vi "WriteScope.vi"(3 "error in (no error)":errorcluster caption="错误输入（无错误）", 4 "本次文件名":string, 5 "report in":refnum<class "NI_report.lvclass"> caption="报表输入") -> (0 "error out":errorcluster caption="错误输出", 2 "report out":refnum<class "NI_report.lvclass"> caption="报表输出")   [LabVIEW 2018]
uses:
  <vilib>/Utility/NIReport.llb/NI_report.lvclass
  ReportItem.ctl
  Init/AllPath.vi
  Reslut.vi
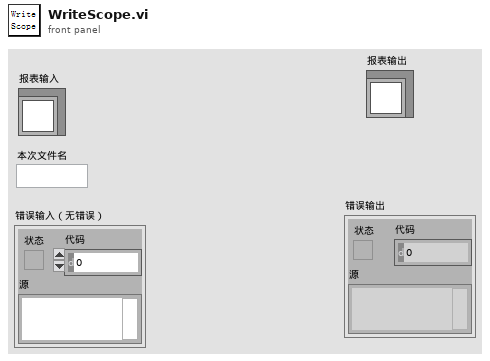
[diagram p1: front panel]
types:
  T1 = typedef "ReportItem.ctl" = enum16{"日期", "激光器编号(Serial)", "功率", "能量", "偏振方向", "偏振度", "脉冲宽度", "脉冲重频", "中心波长", "光谱宽度", "发散角X", "发散角Y", "时间波形路径", "光谱波形路径", "近场图像路径", "远场图像路径", "激光器型号(Type)"}
  T2 = cluster{"波形":waveform(dbl), "脉宽":string, "重频":string, "脉冲宽度Uint":string, "重复频率Uint":string}
  T3 = cluster{"能量/功率":path, " 示波器":path, " 光谱仪":path, "偏振":path, "近远场":cluster{" 近场图片":path, " 远场图片":path, "发散角数据":path}, "参数":path, " 基路径":path, "文件名信息":path, "输出模板路径":path, "输出报告路径":path}
  T4 = typedef "衰减片电机位置枚举器.ctl" = enum16{"0倍", "10倍", "100倍", "1000倍"}
  T5 = cluster{"激光器型号":string, "X":dbl, "Y":dbl, "Z":dbl, "Rotate":dbl, "Pitching":dbl, "DivergeAngle":dbl, "衰减片位置":cluster{"小积分球位置":T4, "偏振仪位置 ":T4, "近场相机位置 ":T4, "远场相机位置":T4}, "Type":string, "Serial":string}
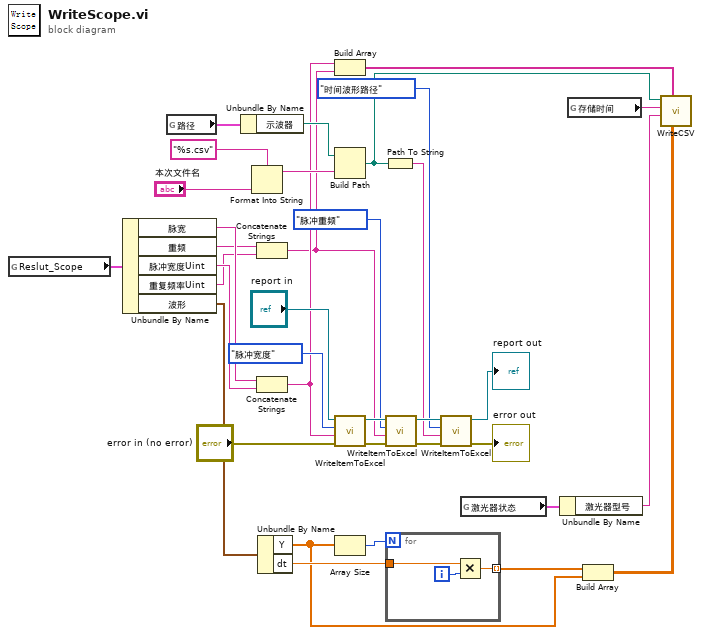
[diagram p0: block diagram]
diagram:
  n1 = global read "Reslut.vi" "Reslut_Scope"() -> (w32:T2)
  n2 = Unbundle By Name(w32) -> ("脉宽"=w28:string, "重频"=w26:string, "脉冲宽度Uint"=w27:string, "重复频率Uint"=w25:string, "波形"=w22:waveform(dbl))
  n3 = global read "AllPath.vi" "路径"() -> (w35:T3)
  n4 = Unbundle By Name(w35) -> ("示波器"=w34:path)
  n5 = Format Into String(format string="%s.csv" ("格式字符串"), "本次文件名") -> (resulting string=w29:string)  [unwired: 2 in, 1 out]
  n6 = Concatenate Strings(w26, w25) -> (w10:string)
  n7 = Concatenate Strings(w28, w27) -> (w11:string)
  n8 = Unbundle By Name(w22) -> ("Y"=w18:dbl[], "dt"=w20:dbl)
  n9 = Build Array(w11, w10) -> (w23:string[])
  n10 = Build Path(base path=w34, name or relative path=w29) -> (appended path=w6:path)
  n11 = call "WriteItemToExcel.vi"("error in (no error)"="error in (no error)", "Data"=w11, "保存类型"=ReportItem."脉冲宽度", "report in"="report in") -> ("error out"=w3:errorcluster, "report out"=w13:refnum<class "NI_report.lvclass">)  [unwired: 6 in]
  n12 = Array Size(array=w18) -> (size(s)=w21:i32)
  n13 = Path To String(path=w6) -> (string=w5:string)
  n14 = call "WriteItemToExcel.vi"("error in (no error)"=w3, "Data"=w10, "保存类型"=ReportItem."脉冲重频", "report in"=w13) -> ("error out"=w2:errorcluster, "report out"=w9:refnum<class "NI_report.lvclass">)  [unwired: 6 in]
  n15 = for {
    N: w21 -> [_]
    tunnel: w20 -> [w37]
    tunnel: [w36] -> w19 mode=indexing
    i -> [w38]
    n16 = Multiply(x=w37, y=w38) -> (x*y=w36:dbl)
  }
  n17 = call "WriteItemToExcel.vi"("error in (no error)"=w2, "Data"=w5, "保存类型"=ReportItem."时间波形路径", "report in"=w9) -> ("error out"=→"error out":errorcluster, "report out"=→"report out":refnum<class "NI_report.lvclass">)  [unwired: 6 in]
  n18 = global read "参数.vi" "激光器状态"() -> (w33:T5)
  n19 = Unbundle By Name(w33) -> ("激光器型号"=w24:string)
  n20 = global read "Reslut.vi" "存储时间"() -> (w16:string)
  n21 = Build Array(w19, w18) -> (w17:dbl[][])
  n22 = call "WriteCSV.vi"("波形"=w17, "通用数据"=w23, "任务编号"=w24, "时间"=w16, "file path (dialog if empty)"=w6) -> ()  [unwired: 7 in]
